vi "JSON Array to Array of Response Objects.vi"(8 "error in (no error)":errorcluster, 11 "JSON Array":string) -> (0 "error out":errorcluster, 3 "Response Objects":string[](array[string]))   [LabVIEW 2019, in "JSON-RPC.lvclass"]
uses:
  JSON-RPC.lvclass
  typedefs/JSON-RPC-Response Object--Cluster.ctl
  lv-venv/lv.lib/vi.lib/addons/_JKI.lib/Serialization/JSON/JKI JSON Serialization.lvlib
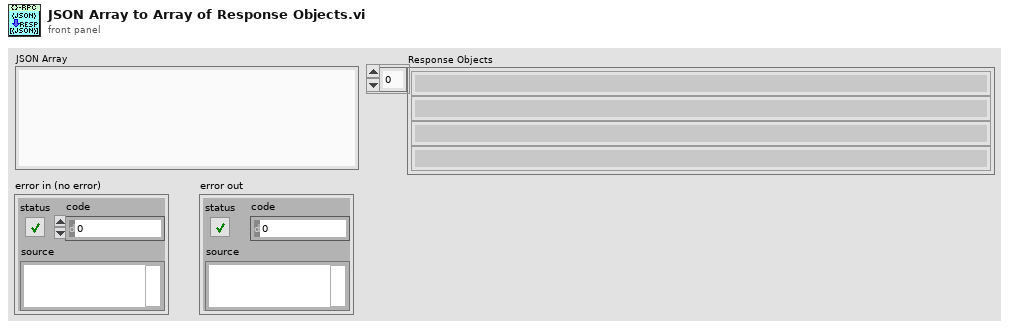
[diagram p1: front panel]
types:
  T1 = typedef "JSON-RPC.lvclass/JSON-RPC-Response Object--Cluster.ctl" = cluster{"jsonrpc":string, "result":variant, "error":variant, "id":string}
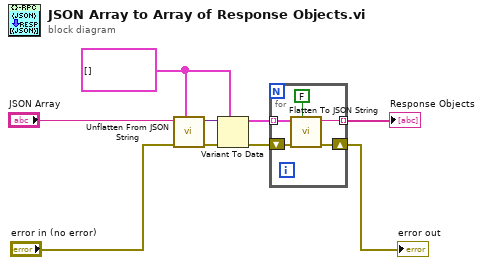
[diagram p0: block diagram]
diagram:
  w6 = T1[] [] ("Array")
  n1 = call "Unflatten From JSON String.vi"("Type and Defaults"=w6, "error in (no error)"="error in (no error)", "JSON String"="JSON Array") -> ("error out"=w8:errorcluster, "Variant"=w7:variant)  [unwired: 7 in]
  n2 = Variant To Data(error in=w8, type=w6, Variant=w7) -> (data=w4:T1[], error out=w3:errorcluster)
  n3 = for {
    tunnel: w4 -> [w14] mode=indexing
    tunnel: [w12] -> w2 mode=indexing
    shift-right: [w11] -> w1
    shift-left: w3 -> [w13]
    n4 = call "Flatten To JSON String.vi"("Multiline (T)"=FALSE, "error in (no error)"=w13, "Variant"=w14) -> ("error out"=w11:errorcluster, "JSON String"=w12:string)  [unwired: 7 in]
  }
  "error out" <- w1
  "Response Objects" <- w2
